vi "Generic command handler.vi"(8 "error in (no error)":errorcluster, 10 "Message in":refnum<class "GenericMessage.lvclass">, 11 "StageSPIM in":refnum<class "StageSPIM.lvclass">) -> (0 "error out":errorcluster, 2 "value":string, 3 "StageSPIM out":refnum<class "StageSPIM.lvclass">)   [LabVIEW 2012, in "StageSPIM.lvclass"]
doc: "The generic_command_handler processes the command 'generic'. Commands which are not part of the predefined list of commands fall under the 'generic' command for special activity."
uses:
  StageSPIM.lvclass
  <vilib>/Distrio/Murmex/GenericMessage/GenericMessage.lvclass
  <vilib>/Distrio/Murmex/Murmex/Murmex.lvclass
  StageSPIM.lvclass/StageSPIM.ctl
  <vilib>/Distrio/Murmex/ProceedMessage/ProceedMessage.lvclass
  <vilib>/Distrio/Murmex/Message/Message.lvclass
panel:
  # "This method is called when the GENERIC\ntrigger is sent. \n\nOverride this method when your component needs to\nrespond to this trigger. \n\nCall parent for proper implementation"
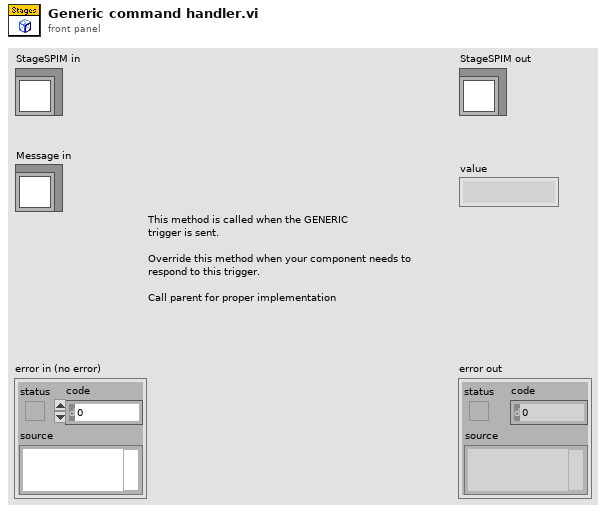
[diagram p1: front panel]
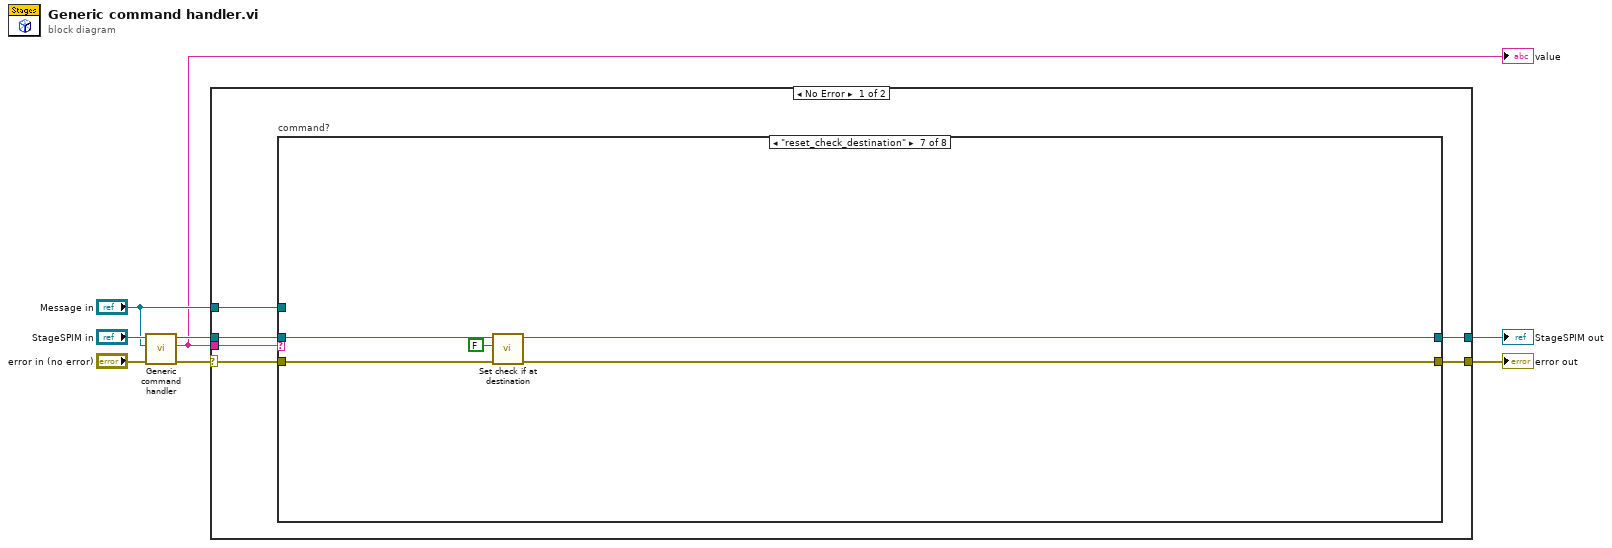
[diagram p0: block diagram]
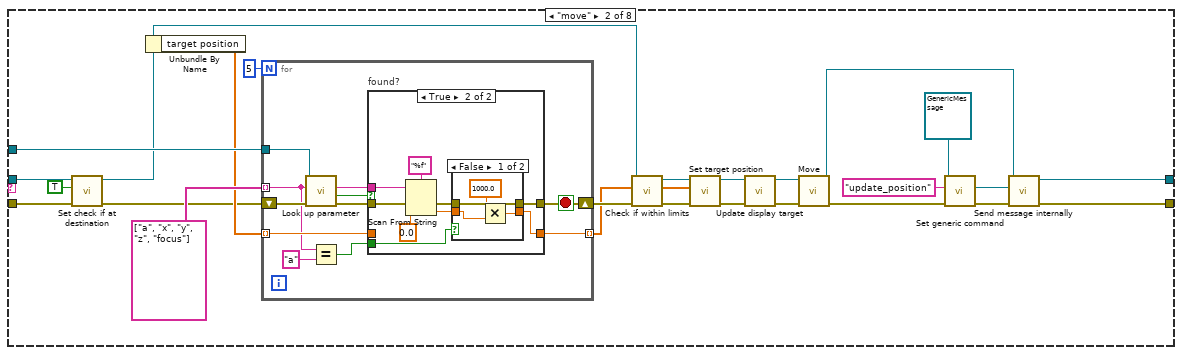
[diagram p3: hidden frame]
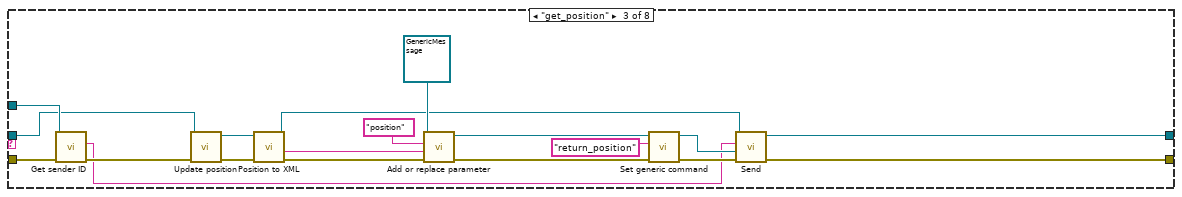
[diagram p6: hidden frame]
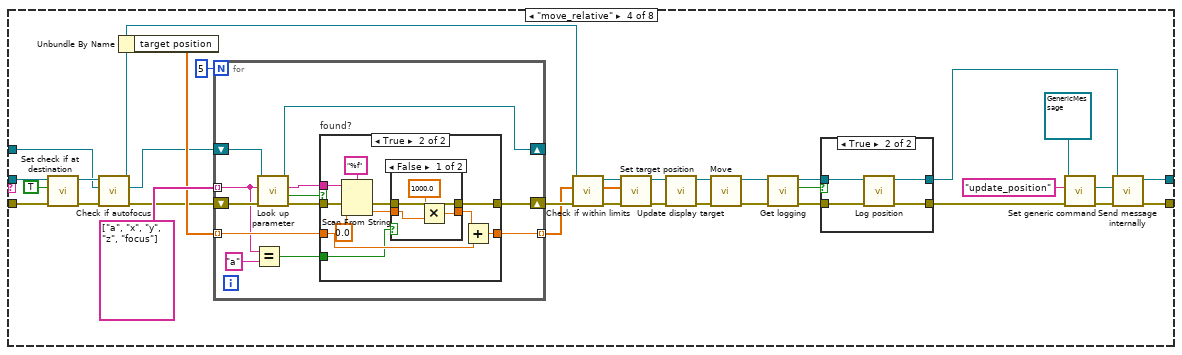
[diagram p7: hidden frame]
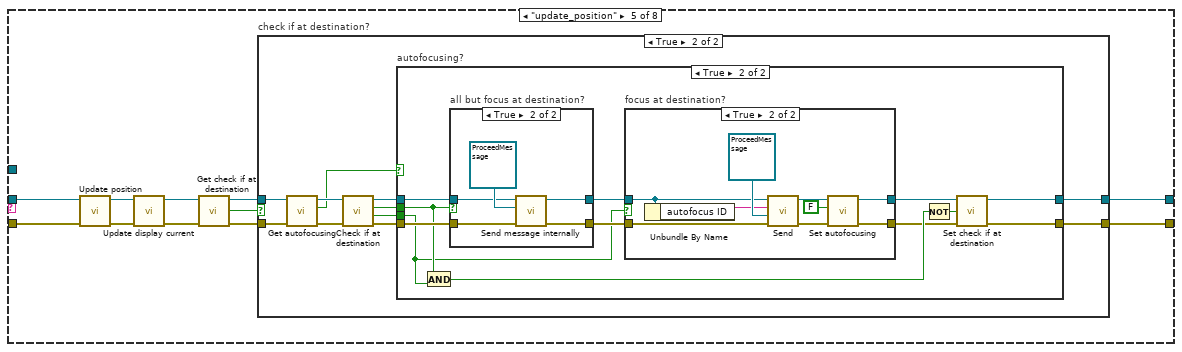
[diagram p11: hidden frame]
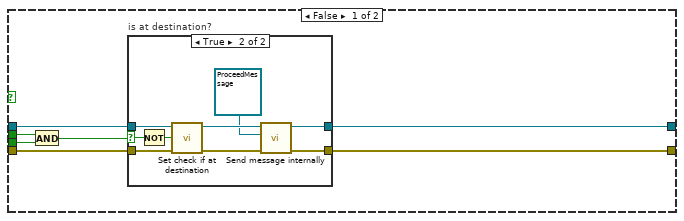
[diagram p13: hidden frame]
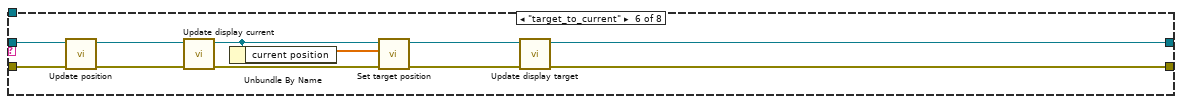
[diagram p17: hidden frame]
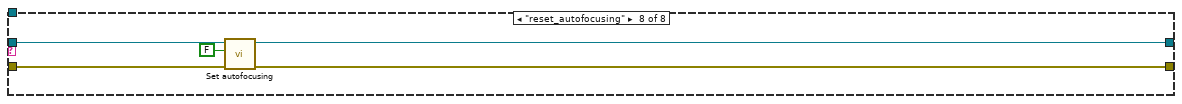
[diagram p18: hidden frame]
diagram:
  n1 = call-parent "Generic command handler.vi"("error in (no error)"="error in (no error)", "Message in"="Message in", "Murmex in"="StageSPIM in") -> ("error out"=w6:errorcluster, "value"=w3:string, "Murmex out"=w5:refnum<class "StageSPIM.lvclass">)  [unwired: 6 in]
  "value" <- w3
  n2 = case shown="No Error" w6 {
    selector: w6 -> [w13 w254]
    tunnel: w3 -> [w14 _]
    tunnel: w5 -> [w12 w255]
    tunnel: "Message in" -> [w11 _]
    tunnel: [w10 w254] -> w2
    tunnel: [w9 w255] -> w1
    frame No Error {
      n3 = case "command?" shown="\"reset_check_destination\"" w14 {
        tunnel: w13 -> [w15 w31 w89 w114 w171 w241 w248 w253]
        tunnel: w12 -> [w16 w33 w75 w115 w170 w240 w247 w252]
        tunnel: w11 -> [_ w38 w88 w97 _ _ _ _]
        tunnel: [w15 w24 w71 w108 w165 w235 w244 w250] -> w10
        tunnel: [w16 w21 w72 w106 w166 w233 w245 w251] -> w9
        frame Default {
        }
        frame "move" {
          n4 = call-dynamic "Set check if at destination.vi"("error in (no error)"=w31, "check if at destination"=TRUE, "StageSPIM in"=w33) -> ("error out"=w30:errorcluster, "StageSPIM out"=w32:refnum<class "StageSPIM.lvclass">)  [unwired: 7 in]
          n5 = Unbundle By Name(w32) -> ("target position"=w35:dbl[])
          n6 = for {
            N: 5 -> [_]
            shift-right: [w46] -> w39
            shift-left: w30 -> [w53]
            tunnel: string[] ["a", "x", "y", "z", "focus"] -> [w44] mode=indexing
            tunnel: w35 -> [w48] mode=indexing
            tunnel: [w47] -> w34 mode=indexing
            tunnel: w38 -> [w49]
            stop <- w46 stop-if-true
            n7 = call <vilib>:"Look up parameter.vi"("error in (no error)"=w53, "name"=w44, "Message in"=w49) -> ("error out"=w52:errorcluster, "found?"=w51:bool, "key"=w50:string)  [unwired: 5 in, 1 out]
            n8 = Equal?(x=w44, y="a") -> (x = y?=w43:bool)
            n9 = case "found?" shown="True" w51 {
              tunnel: w52 -> [w55 w64]
              tunnel: [w55 w59] -> w46
              tunnel: w50 -> [_ w62]
              tunnel: [w54 w57] -> w47
              tunnel: w48 -> [w54 _]
              tunnel: w43 -> [_ w56]
              frame False {
              }
              frame True {
                n10 = Scan From String(format string="%f", input string=w62, error in=w64, default 1=0.0 ("default value 1")) -> (error out=w60:errorcluster, output 1=w58:dbl)  [unwired: 1 in, 2 out]
                n11 = case shown="False" w56 {
                  tunnel: [w68 w70] -> w59
                  tunnel: w60 -> [w68 w70]
                  tunnel: [w67 w69] -> w57
                  tunnel: w58 -> [w66 w69]
                  frame False {
                    n12 = Multiply(x=1000.0, y=w66) -> (x*y=w67:dbl)
                  }
                  frame True {
                  }
                }
              }
            }
          }
          n13 = call-dynamic "Check if within limits.vi"("error in (no error)"=w39, "Position array in"=w34, "StageSPIM in"=w32) -> ("error out"=w41:errorcluster, "Approved postion array"=w40:dbl[], "StageSPIM out"=w42:refnum<class "StageSPIM.lvclass">)  [unwired: 4 in, 2 out]
          n14 = call-dynamic "Set target position.vi"("error in (no error)"=w41, "target position"=w40, "StageSPIM in"=w42) -> ("error out"=w20:errorcluster, "StageSPIM out"=w18:refnum<class "StageSPIM.lvclass">)  [unwired: 7 in]
          n15 = call-dynamic "Update display target.vi"("error in (no error)"=w20, "StageSPIM in"=w18) -> ("error out"=w19:errorcluster, "StageSPIM out"=w17:refnum<class "StageSPIM.lvclass">)  [unwired: 8 in]
          n16 = call-dynamic "Move.vi"("error in (no error)"=w19, "StageSPIM in"=w17) -> ("error out"=w28:errorcluster, "StageSPIM out"=w22:refnum<class "StageSPIM.lvclass">)  [unwired: 8 in]
          n17 = call <vilib>:"Set generic command.vi"("error in (no error)"=w28, "generic command"="update_position", "GenericMessage in"=refnum<class "GenericMessage.lvclass"> refnum ("Distrio Murmex 1.1:GenericMessage")) -> ("error out"=w27:errorcluster, "GenericMessage out"=w23:refnum<class "GenericMessage.lvclass">)  [unwired: 7 in]
          n18 = call <vilib>:"Send message internally.vi"("error in (no error)"=w27, "Message"=w23, "Murmex in"=w22) -> ("error out"=w24:errorcluster, "Murmex out"=w21:refnum<class "StageSPIM.lvclass">)  [unwired: 7 in]
        }
        frame "get_position" {
          n19 = call <vilib>:"Get sender ID.vi"("error in (no error)"=w89, "Message in"=w88) -> ("error out"=w87:errorcluster, "sender"=w83:string)  [unwired: 7 in, 1 out]
          n20 = call-dynamic "Update position.vi"("error in (no error)"=w87, "StageSPIM in"=w75) -> ("error out"=w77:errorcluster, "StageSPIM out"=w74:refnum<class "StageSPIM.lvclass">)  [unwired: 8 in]
          n21 = call-dynamic "Position to XML.vi"("error in (no error)"=w77, "StageSPIM in"=w74) -> ("error out"=w76:errorcluster, "XML string"=w73:string, "StageSPIM out"=w78:refnum<class "StageSPIM.lvclass">)  [unwired: 7 in]
          n22 = call <vilib>:"Add or replace parameter.vi"("error in (no error)"=w76, "value"=w73, "name"="position", "Message in"=refnum<class "GenericMessage.lvclass"> refnum ("Distrio Murmex 1.1:GenericMessage")) -> ("error out"=w81:errorcluster, "Message out"=w80:refnum<class "GenericMessage.lvclass">)  [unwired: 6 in]
          n23 = call <vilib>:"Set generic command.vi"("error in (no error)"=w81, "generic command"="return_position", "GenericMessage in"=w80) -> ("error out"=w85:errorcluster, "GenericMessage out"=w84:refnum<class "GenericMessage.lvclass">)  [unwired: 7 in]
          n24 = call <vilib>:"Send.vi"("error in (no error)"=w85, "Message"=w84, "recipient"=w83, "Murmex in"=w78) -> ("error out"=w71:errorcluster, "Murmex out"=w72:refnum<class "StageSPIM.lvclass">)  [unwired: 6 in]
        }
        frame "move_relative" {
          n25 = call-dynamic "Set check if at destination.vi"("error in (no error)"=w114, "check if at destination"=TRUE, "StageSPIM in"=w115) -> ("error out"=w101:errorcluster, "StageSPIM out"=w99:refnum<class "StageSPIM.lvclass">)  [unwired: 7 in]
          n26 = call-dynamic "Check if autofocus.vi"("error in (no error)"=w101, "Message in"=w97, "StageSPIM in"=w99) -> ("error out"=w100:errorcluster, "Message out"=w96:refnum<class "GenericMessage.lvclass">, "StageSPIM out"=w98:refnum<class "StageSPIM.lvclass">)  [unwired: 6 in]
          n27 = Unbundle By Name(w98) -> ("target position"=w117:dbl[])
          n28 = for {
            N: 5 -> [_]
            shift-right: [w138] -> w120
            shift-left: w100 -> [w141]
            tunnel: string[] ["a", "x", "y", "z", "focus"] -> [w132] mode=indexing
            shift-right: [w135] -> _
            shift-left: w96 -> [w136]
            tunnel: w117 -> [w134] mode=indexing
            tunnel: [w133] -> w116 mode=indexing
            n29 = Equal?(x=w132, y="a") -> (x = y?=w130:bool)
            n30 = call <vilib>:"Look up parameter.vi"("error in (no error)"=w141, "name"=w132, "Message in"=w136) -> ("error out"=w140:errorcluster, "found?"=w139:bool, "key"=w137:string, "Message out"=w135:refnum<class "GenericMessage.lvclass">)  [unwired: 5 in]
            n31 = case "found?" shown="True" w139 {
              tunnel: w140 -> [w143 w154]
              tunnel: [w143 w147] -> w138
              tunnel: w137 -> [_ w152]
              tunnel: [w142 w150] -> w133
              tunnel: w134 -> [w142 w149]
              tunnel: w130 -> [_ w148]
              frame False {
              }
              frame True {
                n32 = Scan From String(format string="%f", input string=w152, error in=w154, default 1=0.0 ("default value 1")) -> (error out=w146:errorcluster, output 1=w144:dbl)  [unwired: 1 in, 2 out]
                n33 = case shown="False" w148 {
                  tunnel: [w158 w160] -> w147
                  tunnel: w146 -> [w158 w160]
                  tunnel: [w157 w159] -> w145
                  tunnel: w144 -> [w156 w159]
                  frame False {
                    n34 = Multiply(x=1000.0, y=w156) -> (x*y=w157:dbl)
                  }
                  frame True {
                  }
                }
                n35 = Add(x=w145, y=w149) -> (x+y=w150:dbl)
              }
            }
          }
          n36 = call-dynamic "Check if within limits.vi"("error in (no error)"=w120, "Position array in"=w116, "StageSPIM in"=w98) -> ("error out"=w122:errorcluster, "Approved postion array"=w121:dbl[], "StageSPIM out"=w123:refnum<class "StageSPIM.lvclass">)  [unwired: 4 in, 2 out]
          n37 = call-dynamic "Set target position.vi"("error in (no error)"=w122, "target position"=w121, "StageSPIM in"=w123) -> ("error out"=w105:errorcluster, "StageSPIM out"=w102:refnum<class "StageSPIM.lvclass">)  [unwired: 7 in]
          n38 = call-dynamic "Update display target.vi"("error in (no error)"=w105, "StageSPIM in"=w102) -> ("error out"=w104:errorcluster, "StageSPIM out"=w103:refnum<class "StageSPIM.lvclass">)  [unwired: 8 in]
          n39 = call-dynamic "Move.vi"("error in (no error)"=w104, "StageSPIM in"=w103) -> ("error out"=w112:errorcluster, "StageSPIM out"=w91:refnum<class "StageSPIM.lvclass">)  [unwired: 8 in]
          n40 = call-dynamic "Get logging.vi"("error in (no error)"=w112, "StageSPIM in"=w91) -> ("error out"=w94:errorcluster, "logging?"=w95:bool, "StageSPIM out"=w93:refnum<class "StageSPIM.lvclass">)  [unwired: 7 in]
          n41 = case shown="True" w95 {
            tunnel: w94 -> [w125 w129]
            tunnel: w93 -> [w124 w128]
            tunnel: [w125 w126] -> w92
            tunnel: [w124 w127] -> w90
            frame False {
            }
            frame True {
              n42 = call-dynamic "Log position.vi"("error in (no error)"=w129, "StageSPIM in"=w128) -> ("error out"=w126:errorcluster, "StageSPIM out"=w127:refnum<class "StageSPIM.lvclass">)  [unwired: 8 in]
            }
          }
          n43 = call <vilib>:"Set generic command.vi"("error in (no error)"=w92, "generic command"="update_position", "GenericMessage in"=refnum<class "GenericMessage.lvclass"> refnum ("Distrio Murmex 1.1:GenericMessage")) -> ("error out"=w111:errorcluster, "GenericMessage out"=w107:refnum<class "GenericMessage.lvclass">)  [unwired: 7 in]
          n44 = call <vilib>:"Send message internally.vi"("error in (no error)"=w111, "Message"=w107, "Murmex in"=w90) -> ("error out"=w108:errorcluster, "Murmex out"=w106:refnum<class "StageSPIM.lvclass">)  [unwired: 7 in]
        }
        frame "update_position" {
          n45 = call-dynamic "Update position.vi"("error in (no error)"=w171, "StageSPIM in"=w170) -> ("error out"=w164:errorcluster, "StageSPIM out"=w162:refnum<class "StageSPIM.lvclass">)  [unwired: 8 in]
          n46 = call-dynamic "Update display current.vi"("error in (no error)"=w164, "StageSPIM in"=w162) -> ("error out"=w163:errorcluster, "StageSPIM out"=w161:refnum<class "StageSPIM.lvclass">)  [unwired: 8 in]
          n47 = call-dynamic "Get check if at destination.vi"("error in (no error)"=w163, "StageSPIM in"=w161) -> ("error out"=w168:errorcluster, "check if at destination"=w169:bool, "StageSPIM out"=w167:refnum<class "StageSPIM.lvclass">)  [unwired: 7 in]
          n48 = case "check if at destination?" shown="True" w169 {
            tunnel: w168 -> [w173 w179]
            tunnel: w167 -> [w172 w177]
            tunnel: [w172 w181] -> w166
            tunnel: [w173 w180] -> w165
            frame False {
            }
            frame True {
              n49 = call-dynamic "Get autofocusing.vi"("error in (no error)"=w179, "StageSPIM in"=w177) -> ("error out"=w178:errorcluster, "autofocusing?"=w175:bool, "StageSPIM out"=w176:refnum<class "StageSPIM.lvclass">)  [unwired: 7 in]
              n50 = call-dynamic "Check if at destination.vi"("error in (no error)"=w178, "StageSPIM in"=w176) -> ("error out"=w183:errorcluster, "focus at destination?"=w174:bool, "at destination? (all but focus)"=w184:bool, "StageSPIM out"=w182:refnum<class "StageSPIM.lvclass">)  [unwired: 6 in]
              n51 = case "autofocusing?" shown="True" w175 {
                tunnel: w184 -> [w187 w210]
                tunnel: w183 -> [w191 w214]
                tunnel: w182 -> [w190 w213]
                tunnel: [w189 w203] -> w181
                tunnel: [w188 w205] -> w180
                tunnel: w174 -> [w186 w209]
                frame False {
                  n52 = And(x=w187, y=w186) -> (x .and. y?=w185:bool)
                  n53 = case "is at destination?" shown="True" w185 {
                    selector: w185 -> [_ w201]
                    tunnel: w191 -> [w193 w202]
                    tunnel: w190 -> [w192 w199]
                    tunnel: [w193 w195] -> w188
                    tunnel: [w192 w194] -> w189
                    frame False {
                    }
                    frame True {
                      n54 = Not(x=w201) -> (.not. x?=w200:bool)
                      n55 = call-dynamic "Set check if at destination.vi"("error in (no error)"=w202, "check if at destination"=w200, "StageSPIM in"=w199) -> ("error out"=w198:errorcluster, "StageSPIM out"=w197:refnum<class "StageSPIM.lvclass">)  [unwired: 7 in]
                      n56 = call <vilib>:"Send message internally.vi"("error in (no error)"=w198, "Message"=refnum<class "ProceedMessage.lvclass"> refnum ("Distrio Murmex 1.1:ProceedMessage"), "Murmex in"=w197) -> ("error out"=w195:errorcluster, "Murmex out"=w194:refnum<class "StageSPIM.lvclass">)  [unwired: 7 in]
                    }
                  }
                }
                frame True {
                  n57 = And(x=w210, y=w209) -> (x .and. y?=w207:bool)
                  n58 = case "all but focus at destination?" shown="True" w210 {
                    tunnel: w214 -> [w227 w228]
                    tunnel: w213 -> [w226 w229]
                    tunnel: [w227 w231] -> w211
                    tunnel: [w226 w230] -> w212
                    frame False {
                    }
                    frame True {
                      n59 = call <vilib>:"Send message internally.vi"("error in (no error)"=w228, "Message"=refnum<class "ProceedMessage.lvclass"> refnum ("Distrio Murmex 1.1:ProceedMessage"), "Murmex in"=w229) -> ("error out"=w231:errorcluster, "Murmex out"=w230:refnum<class "StageSPIM.lvclass">)  [unwired: 7 in]
                    }
                  }
                  n60 = case "focus at destination?" shown="True" w209 {
                    tunnel: w211 -> [w216 w225]
                    tunnel: w212 -> [w215 w222]
                    tunnel: [w216 w220] -> w206
                    tunnel: [w215 w218] -> w204
                    frame False {
                    }
                    frame True {
                      n61 = Unbundle By Name(w222) -> ("autofocus ID"=w221:string)
                      n62 = call <vilib>:"Send.vi"("error in (no error)"=w225, "Message"=refnum<class "ProceedMessage.lvclass"> refnum ("Distrio Murmex 1.1:ProceedMessage"), "recipient"=w221, "Murmex in"=w222) -> ("error out"=w224:errorcluster, "Murmex out"=w219:refnum<class "StageSPIM.lvclass">)  [unwired: 6 in]
                      n63 = call-dynamic "Set autofocusing.vi"("error in (no error)"=w224, "autofocusing?"=FALSE, "StageSPIM in"=w219) -> ("error out"=w220:errorcluster, "StageSPIM out"=w218:refnum<class "StageSPIM.lvclass">)  [unwired: 7 in]
                    }
                  }
                  n64 = Not(x=w207) -> (.not. x?=w208:bool)
                  n65 = call-dynamic "Set check if at destination.vi"("error in (no error)"=w206, "check if at destination"=w208, "StageSPIM in"=w204) -> ("error out"=w205:errorcluster, "StageSPIM out"=w203:refnum<class "StageSPIM.lvclass">)  [unwired: 7 in]
                }
              }
            }
          }
        }
        frame "target_to_current" {
          n66 = call-dynamic "Update position.vi"("error in (no error)"=w241, "StageSPIM in"=w240) -> ("error out"=w243:errorcluster, "StageSPIM out"=w242:refnum<class "StageSPIM.lvclass">)  [unwired: 8 in]
          n67 = call-dynamic "Update display current.vi"("error in (no error)"=w243, "StageSPIM in"=w242) -> ("error out"=w238:errorcluster, "StageSPIM out"=w239:refnum<class "StageSPIM.lvclass">)  [unwired: 8 in]
          n68 = Unbundle By Name(w239) -> ("current position"=w237:dbl[])
          n69 = call-dynamic "Set target position.vi"("error in (no error)"=w238, "target position"=w237, "StageSPIM in"=w239) -> ("error out"=w236:errorcluster, "StageSPIM out"=w234:refnum<class "StageSPIM.lvclass">)  [unwired: 7 in]
          n70 = call-dynamic "Update display target.vi"("error in (no error)"=w236, "StageSPIM in"=w234) -> ("error out"=w235:errorcluster, "StageSPIM out"=w233:refnum<class "StageSPIM.lvclass">)  [unwired: 8 in]
        }
        frame "reset_check_destination" {
          n71 = call-dynamic "Set check if at destination.vi"("error in (no error)"=w248, "check if at destination"=FALSE, "StageSPIM in"=w247) -> ("error out"=w244:errorcluster, "StageSPIM out"=w245:refnum<class "StageSPIM.lvclass">)  [unwired: 7 in]
        }
        frame "reset_autofocusing" {
          n72 = call-dynamic "Set autofocusing.vi"("error in (no error)"=w253, "autofocusing?"=FALSE ("check if at destination"), "StageSPIM in"=w252) -> ("error out"=w250:errorcluster, "StageSPIM out"=w251:refnum<class "StageSPIM.lvclass">)  [unwired: 7 in]
        }
      }
    }
    frame Error {
    }
  }
  "error out" <- w2
  "StageSPIM out" <- w1
